vi "Analyze all images in tdms file.vi"(11 "file path":path) -> (3 "Intensity Graph":u16[][](graph))   [LabVIEW 2020]
uses:
  <userlib>/_MGI/File/Spreadsheet/MGI Write Spreadsheet Behavior Enum.ctl
panel:
  out "image #":i32
  in  "stop":bool
  out "# pix per image":i32
  out "number images":i32
  out "channel name out":string
  out "data 3":i32
  out "property names":string[](array[string])
  out "property values":variant[](array[variant])
  out "channel names":string[](array[string])
  out "found 2":bool
  out "found":bool
  out "width":i32
  out "size(s)":i32
  out "time to read":u32
  out "data":u16[](array[numeric])
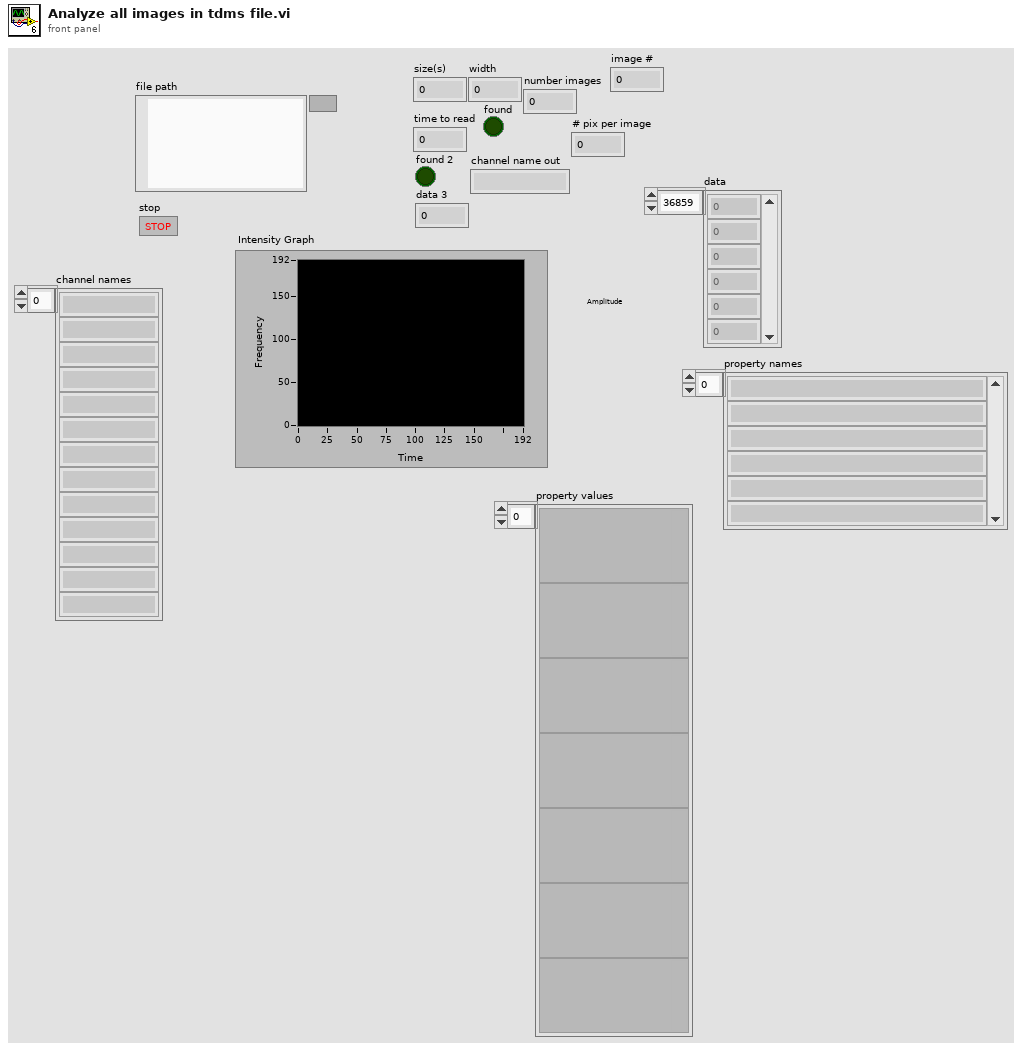
[diagram p1: front panel]
types:
  T1 = typedef "MGI Write Spreadsheet Behavior Enum.ctl" = enum16{"Append data", "Append headers and data", "Overwrite"}
  T2 = enum16{"open", "open or create", "create or replace", "create", "open (read-only)"}
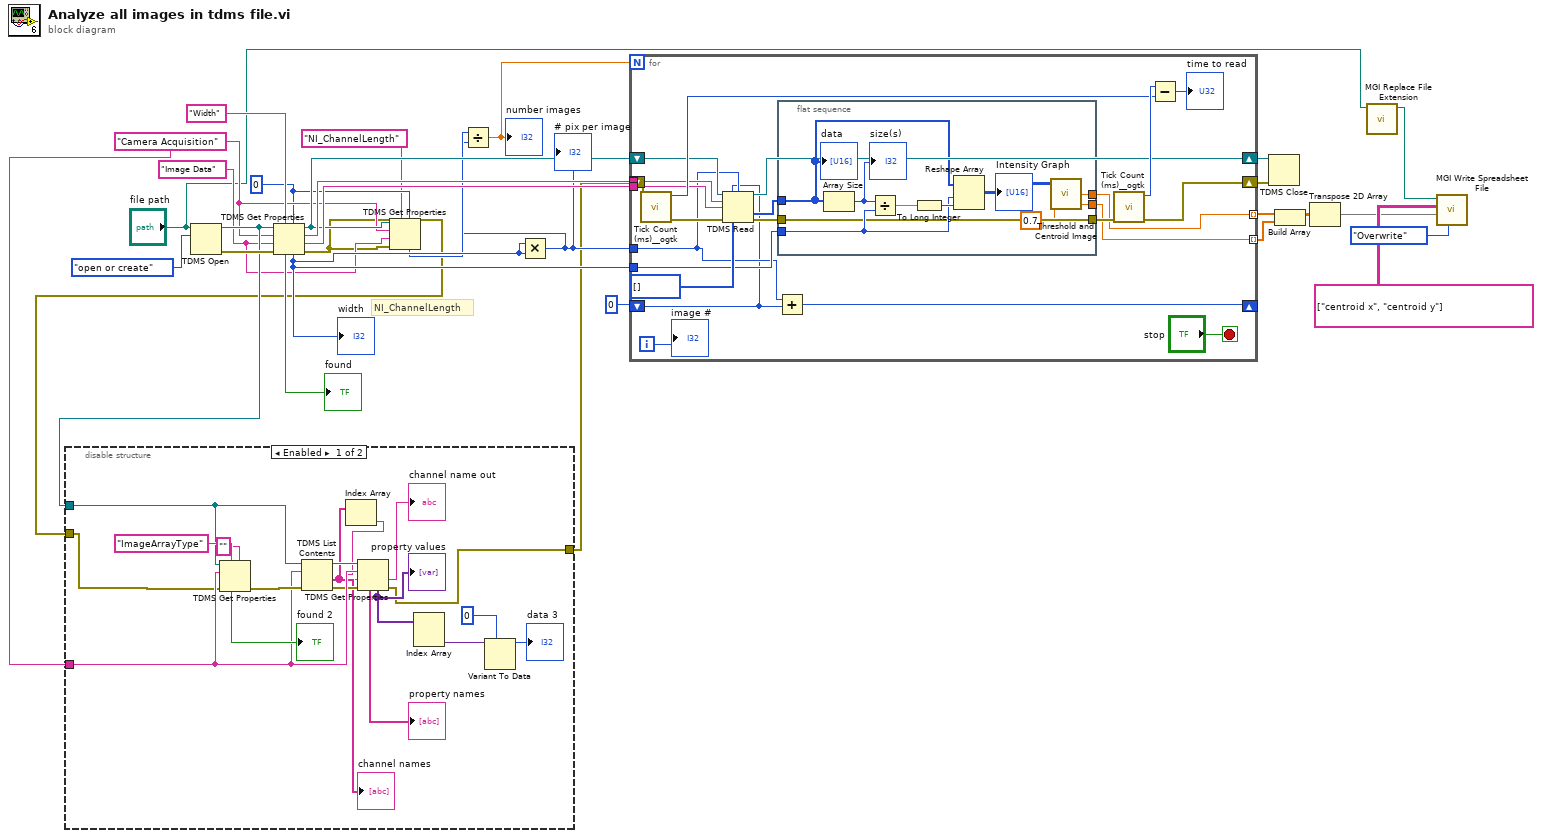
[diagram p0: block diagram]
diagram:
  w17 = 0 ("x")
  w19 = "Camera Acquisition" ("group name in")
  w18 = "Image Data" ("channel name(s) in")
  # "NI_ChannelLength"
  n1 = TDMS Open(10:T2."open or create" ("operation (0:open)"), 11:"file path") -> (0:w27:errorcluster, 3:w21:refnum<k34>)  [unwired: 5 in]
  n2 = TDMS Get Properties(5:w17, 7:"Width", 8:w27, 9:w18, 10:w19, 11:w21) -> (0:w13:errorcluster, 1:w22:string, 2:w23:string, 3:w20:refnum<k34>, 4:w24:i32, 6:→"found":bool)
  "width" <- w24
  n3 = disable-structure shown="Enabled" {
    disable-tunnel: w21 -> [w44 _]
    disable-tunnel: [w35 _] -> w12
    disable-tunnel: w19 -> [w34 _]
    disable-tunnel: w13 -> [w30 _]
    frame Enabled {
      n4 = TDMS Get Properties(5:"" ("data type"), 7:"ImageArrayType", 8:w30, 10:w34, 11:w44) -> (0:w43:errorcluster, 6:→"found 2":bool)  [unwired: 1 in, 4 out]
      n5 = TDMS List Contents(4:w43, 6:w34, 7:w44) -> (0:w33:errorcluster, 1:w32:string[], 3:w42:refnum<k34>)  [unwired: 1 out]
      "channel names" <- w32
      n6 = Index Array(array=w32) -> (element=w31:string)  [unwired: 1 in]
      n7 = TDMS Get Properties(8:w33, 9:w31, 10:w34, 11:w42) -> (0:w35:errorcluster, 1:→"channel name out":string, 4:w40:variant[], 6:→"property names":string[])  [unwired: 2 in, 2 out]
      "property values" <- w40
      n8 = Index Array(array=w40) -> (element #2=w36:variant)  [unwired: 2 in, 1 out]
      n9 = Variant To Data(type=0, Variant=w36) -> (data=→"data 3":i32)  [unwired: 1 in, 1 out]
    }
    frame Disabled {
    }
  }
  n10 = TDMS Get Properties(5:w17, 7:"NI_ChannelLength" ("property name"), 8:w13, 9:w18, 10:w19, 11:w20) -> (4:w15:i32)  [unwired: 5 out]
  n11 = Multiply(x=w24, y=w24) -> (x*y=w14:i32)
  "# pix per image" <- w14
  n12 = Divide(x=w15, y=w14) -> (x/y=w9:dbl)
  "number images" <- w9
  n13 = for {
    N: w9 -> [_]
    tunnel: w24 -> [w61]
    tunnel: w23 -> [w60]
    tunnel: w22 -> [w59]
    tunnel: w14 -> [w54]
    shift-right: [w65] -> w28
    shift-left: w20 -> [w57]
    shift-right: [w55] -> w11
    shift-left: w12 -> [w56]
    shift-right: [w53] -> _
    shift-left: 0 ("type") -> [w52]
    tunnel: [w49] -> w8 mode=indexing
    tunnel: [w48] -> w7 mode=indexing
    i -> [w50]
    stop <- "stop" stop-if-true
    n14 = call <userlib>:"Tick Count (ms)__ogtk.vi"("error in (no error)"=w56) -> ("error out"=w68:errorcluster, "millisecond timer value"=w66:u32)  [unwired: 9 in]
    n15 = TDMS Read(0:w57, 1:w52, 2:w54, 5:w60, 7:w59, 11:w68, 12:u16[] [] ("output array")) -> (4:w65:refnum<k34>, 10:w63:u16[], 15:w58:errorcluster)  [unwired: 1 in, 3 out]
    n16 = Add(x=w54, y=w52) -> (x+y=w53:i32)
    n17 = flat-sequence {
      tunnel: w63 -> [w79]
      tunnel: w61 -> [w75]
      tunnel: w58 -> [w74]
      tunnel: [w74] -> w62
      tunnel: [w71] -> w49
      tunnel: [w70] -> w48
      frame #0 {
        n18 = Array Size(array=w79) -> (size(s)=w78:i32)
        "size(s)" <- w78
        n19 = Divide(x=w78, y=w75) -> (x/y=w77:dbl)
        n20 = To Long Integer(number=w77) -> (32bit integer=w76:i32)
        n21 = Reshape Array(w79, w75, w76) -> (w73:u16[][])
        "Intensity Graph" <- w73
        n22 = call "Threshold and Centroid Image.vi"("Raw Image"=w73, "Threshold or Threshold Fraction*"=0.7) -> ("x0"=w71:dbl, "y0"=w70:dbl)  [unwired: 2 in, 4 out]
        "data" <- w79
      }
    }
    n23 = call <userlib>:"Tick Count (ms)__ogtk.vi"("error in (no error)"=w62) -> ("error out"=w55:errorcluster, "millisecond timer value"=w67:u32)  [unwired: 9 in]
    n24 = Subtract(x=w67, y=w66) -> (x-y=→"time to read":u32)
    "image #" <- w50
  }
  n25 = TDMS Close(8:w11, 11:w28) -> ()  [unwired: 2 out]
  n26 = Build Array(w8, w7) -> (w6:dbl[][])
  n27 = Transpose 2D Array(2D array=w6) -> (transposed array=w1:dbl[][])
  n28 = call <userlib>:"MGI Replace File Extension.vi"("Path In"="file path") -> ("Path Out"=w3:path)  [unwired: 9 in, 1 out]
  n29 = call <userlib>:"MGI Write Spreadsheet File.vi"("Existing File Behavior"=MGI_Write_Spreadsheet_Behavior_Enum."Overwrite", "Data[row][col]"=w1, "Header Lines[row][col]"=string[][] [["centroid x", "centroid y"]], "Path"=w3) -> ()  [unwired: 4 in, 4 out]
